vi "PAN_ParseForCmdSet.vi"(7 "defcmdset":string="NATIVE", 10 "cmd in":string) -> (1 "cmdset":string, 2 "cmd out":string)   [LabVIEW 2016]
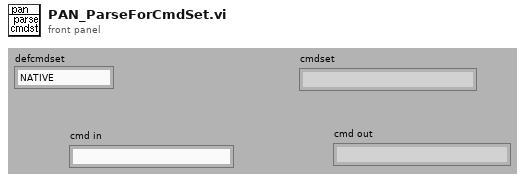
[diagram p1: front panel]
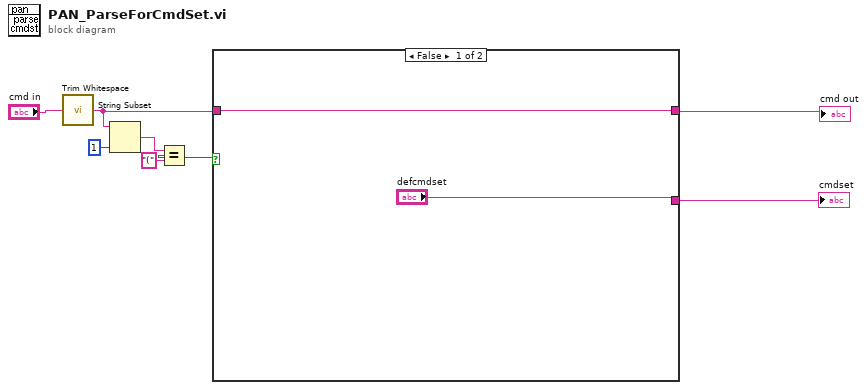
[diagram p0: block diagram]
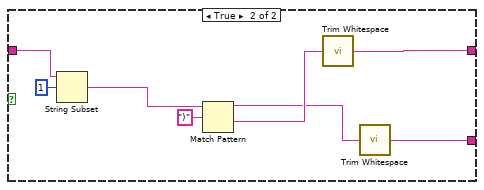
[diagram p2: hidden frame]
diagram:
  n1 = call <vilib>:"Trim Whitespace.vi"("string"="cmd in") -> ("trimmed string"=w1:string)  [unwired: 1 in]
  n2 = String Subset(string=w1, length (rest)=1 ("length (rest)")) -> (substring=w7:string)  [unwired: 1 out]
  n3 = Equal?(x=w7, y="(") -> (x = y?=w5:bool)
  n4 = case shown="False" w5 {
    tunnel: w1 -> [w10 w14]
    tunnel: [w10 w12] -> w3
    tunnel: ["defcmdset" w11] -> w2
    frame False {
    }
    frame True {
      n5 = String Subset(string=w14, offset (0)=1) -> (substring=w13:string)  [unwired: 1 out]
      n6 = Match Pattern(string=w13, regular expression=")") -> (before substring=w16:string, after substring=w17:string)  [unwired: 3 out]
      n7 = call <vilib>:"Trim Whitespace.vi"("string"=w17) -> ("trimmed string"=w12:string)  [unwired: 1 in]
      n8 = call <vilib>:"Trim Whitespace.vi"("string"=w16) -> ("trimmed string"=w11:string)  [unwired: 1 in]
    }
  }
  "cmd out" <- w3
  "cmdset" <- w2
